vi "Create OneOf Field Accessors.vi"(8 "error in (no error)":errorcluster, 10 "Message parameters":T1[](array[typedef]), 11 "Library in":refnum<vi>) -> (0 "error out":errorcluster, 3 "Library out":refnum<vi>)   [LabVIEW 2019, in "gRPC Template Creation Utility.lvlib"]
uses:
  gRPC Template Creation Utility.lvlib
  TypeDefs/Message Element Type.ctl
  TypeDefs/Message Element Metadata (Scripting).ctl
  TypeDefs/Message Metadata (Scripting).ctl
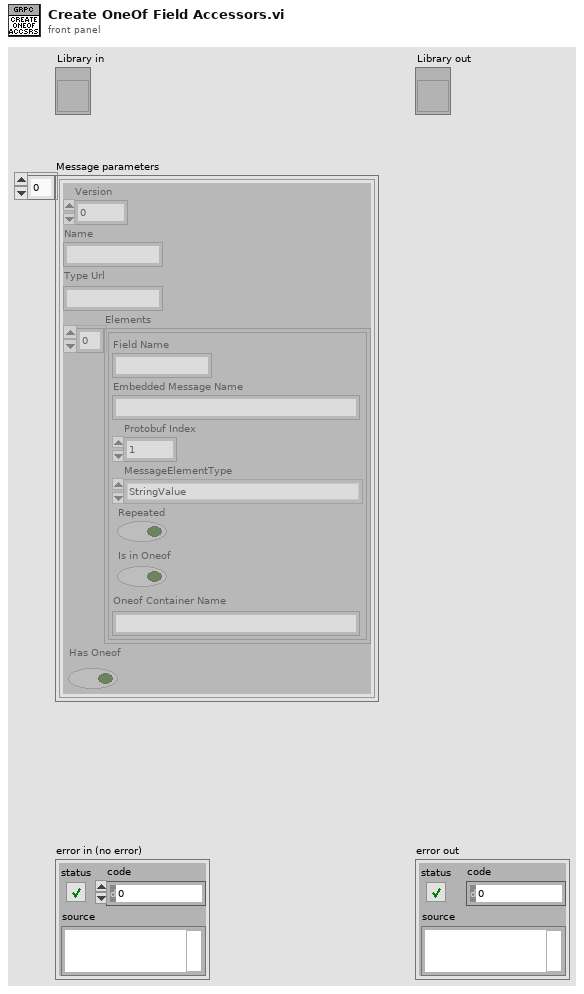
[diagram p1: front panel]
types:
  T1 = typedef "gRPC Template Creation Utility.lvlib/Message Metadata (Scripting).ctl" = cluster{"Version":i32, "Name":string, "Type Url":string, "Elements":T2[], "Has Oneof":bool}
  T2 = typedef "gRPC Template Creation Utility.lvlib/Message Element Metadata (Scripting).ctl" = cluster{"Field Name":string, "Embedded Message Name":string, "Protobuf Index":i32, "MessageElementType":T3, "Repeated":bool, "Is in Oneof":bool, "Oneof Container Name":string}
  T3 = typedef "gRPC Template Creation Utility.lvlib/Message Element Type.ctl" = enum32{"Int32Value", "FloatValue", "DoubleValue", "BoolValue", "StringValue", "MessageValue", "Int64Value", "UInt32Value", "UInt64Value", "EnumValue", "Bytes", "Fixed64", "Fixed32", "SFixed64", "SFixed32", "SInt64", "SInt32"}
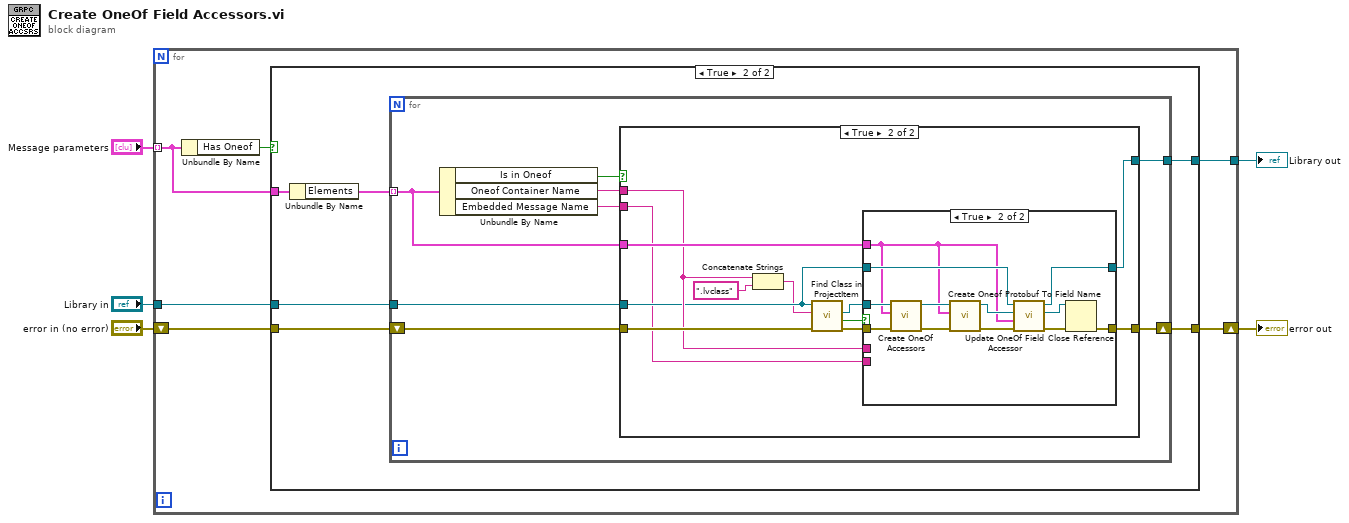
[diagram p0: block diagram]
diagram:
  n1 = for {
    tunnel: "Message parameters" -> [w10] mode=indexing
    tunnel: "Library in" -> [w8]
    shift-right: [w7] -> w2
    shift-left: "error in (no error)" -> [w9]
    tunnel: [w6] -> w1
    n2 = Unbundle By Name(w10) -> ("Has Oneof"=w11:bool)
    n3 = case shown="True" w11 {
      tunnel: w10 -> [_ w19]
      tunnel: w9 -> [w13 w17]
      tunnel: w8 -> [w12 w16]
      tunnel: [w13 w15] -> w7
      tunnel: [w12 w14] -> w6
      frame False {
      }
      frame True {
        n4 = Unbundle By Name(w19) -> ("Elements"=w18:T2[])
        n5 = for {
          tunnel: w18 -> [w27] mode=indexing
          tunnel: w16 -> [w25]
          shift-right: [w24] -> w15
          shift-left: w17 -> [w26]
          tunnel: [w23] -> w14
          n6 = Unbundle By Name(w27) -> ("Is in Oneof"=w22:bool, "Oneof Container Name"=w21:string, "Embedded Message Name"=w20:string)
          n7 = case shown="True" w22 {
            tunnel: w26 -> [w28 w39]
            tunnel: w27 -> [_ w41]
            tunnel: [w28 w40] -> w24
            tunnel: [w29 w30] -> w23
            tunnel: w21 -> [_ w37]
            tunnel: w25 -> [w29 w34]
            tunnel: w20 -> [_ w31]
            frame False {
            }
            frame True {
              n8 = Concatenate Strings(w37, ".lvclass" ("string")) -> (w33:string)
              n9 = call "Find Class in ProjectItem.vi"("error in (no error)"=w39, "Class Name"=w33, "ProjectItem in"=w34) -> ("error out"=w38:errorcluster, "Found?"=w36:bool, "LVClass out"=w35:refnum<vi>)  [unwired: 5 in, 1 out]
              n10 = case shown="True" w36 {
                tunnel: w41 -> [_ w48]
                tunnel: [w43 w45] -> w40
                tunnel: w38 -> [w43 w54]
                tunnel: w37 -> [_ _]
                tunnel: w35 -> [_ w53]
                tunnel: w34 -> [w42 w50]
                tunnel: w31 -> [_ _]
                tunnel: [w42 w44] -> w30
                frame False {
                }
                frame True {
                  n11 = call "Create OneOf Accessors.vi"("error in (no error)"=w54, "MessageElementMetadata"=w48, "Oneof Class Ref In"=w53) -> ("error out"=w55:errorcluster, "Oneof Class Ref Out"=w49:refnum<vi>)  [unwired: 7 in]
                  n12 = call "Create Oneof Protobuf To Field Name.vi"("error in (no error)"=w55, "message element metadata"=w48, "class in"=w49) -> ("error out"=w52:errorcluster, "class out"=w51:refnum<vi>)  [unwired: 7 in]
                  n13 = call "Update OneOf Field Accessor.vi"("error in (no error)"=w52, "message element metadata"=w48, "class in"=w51, "library in"=w50) -> ("error out"=w47:errorcluster, "class out"=w46:refnum<vi>, "library out"=w44:refnum<vi>)  [unwired: 5 in]
                  n14 = Close Reference(reference=w46, error in (no error)=w47) -> (error out=w45:errorcluster)
                }
              }
            }
          }
        }
      }
    }
  }
  "error out" <- w2
  "Library out" <- w1
